vi "FTW-Listener-Destroy.vi"(0 "FTW-Listener-LVQ In":refnum<class "FTW-Listener-LVQ.lvclass">, 11 "error in":errorcluster) -> (15 "error out":errorcluster)   [LabVIEW 2013, in "FTW-Listener-LVQ.lvclass"]
uses:
  FTW-Listener-LVQ.lvclass
  FTW-Listener-LVQ.lvclass/FTW-Listener-LVQ.ctl
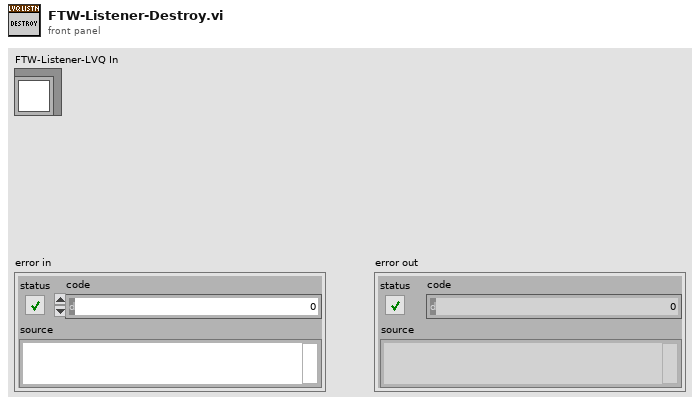
[diagram p1: front panel]
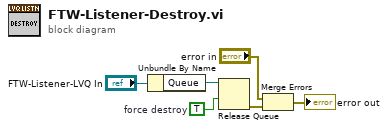
[diagram p0: block diagram]
diagram:
  w1 = TRUE  # force destroy
  n1 = Unbundle By Name("FTW-Listener-LVQ In") -> ("Queue"=w4:refnum<queue>)
  n2 = Release Queue(queue=w4, force destroy? (F)=w1) -> (error out=w2:errorcluster)  [unwired: 1 in, 2 out]
  n3 = Merge Errors("error in", w2) -> (→"error out":errorcluster)
